vi "Do.vi"(8 "error in (no error)":errorcluster, 10 "Actor in":refnum<class "Actor.lvclass">, 11 "Connection Msg":refnum<class "Connection Msg.lvclass">) -> (0 "error out":errorcluster, 2 "Actor out":refnum<class "Actor.lvclass">)   [LabVIEW 2025, in "PLC_Abstr.lvlib" / "Connection Msg.lvclass"]
doc: "This VI delivers the message to the actor by calling the appropriate method(s) on the actor."
uses:
  Connection Msg.lvclass
  <vilib>/ActorFramework/Actor/Actor.lvclass
  Connection Msg.lvclass/Connection Msg.ctl
  PLC_Abstr/PLC_Abstr.lvclass
  9ef47adc-f318-494c-9b8b-6df3216d6863.vi
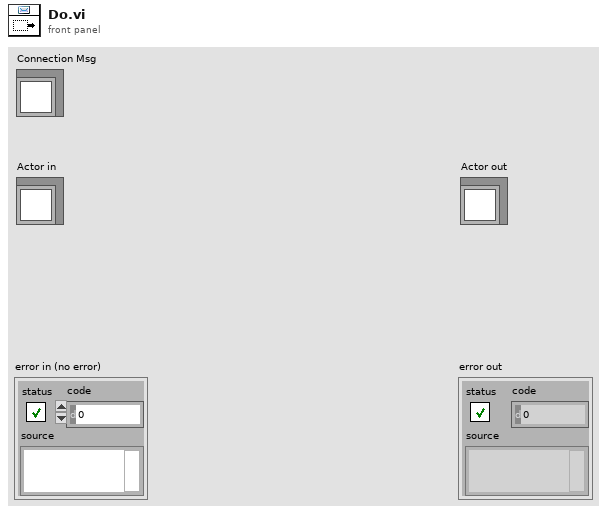
[diagram p1: front panel]
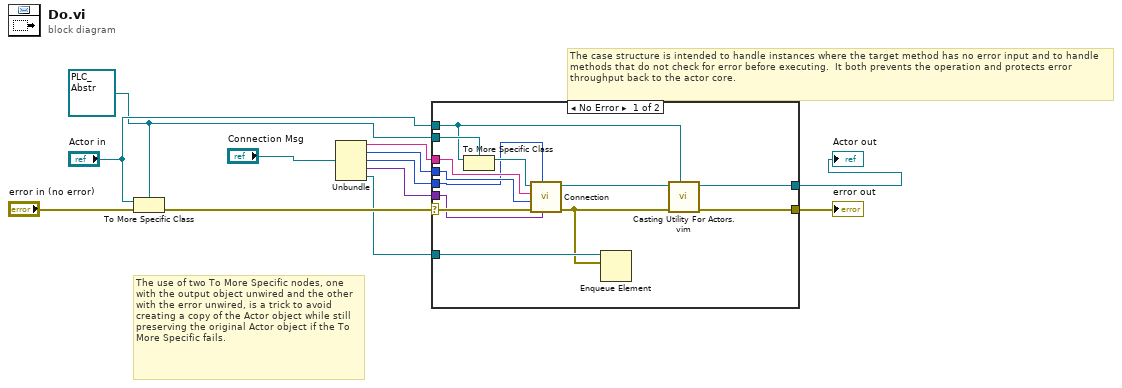
[diagram p0: block diagram]
diagram:
  w6 = refnum<class "PLC_Abstr.lvclass"> refnum ("Actor in")
  # "The use of two To More Specific nodes, one with the output object unwired and the other with the error unwired, is a trick to avoid creating a copy of the Actor object while still preserving the original Actor object if the To More Specific fails."
  # "The case structure is intended to handle instances where the target method has no error input and to handle methods that do not check for error before executing.  It both prevents the operation and protects error throughput back to the actor core."
  n1 = To More Specific Class(target class=w6, reference="Actor in", error in="error in (no error)") -> (error out=w10:errorcluster)  [unwired: 1 out]
  n2 = Unbundle("Connection Msg") -> (w5:string, w4:u16, w3:i32, w2:variant, w1:refnum<queue>)
  n3 = case shown="No Error" w10 {
    selector: w10 -> [w25 w27]
    tunnel: [w19 w27] -> w9
    tunnel: [w20 w26] -> w8
    tunnel: "Actor in" -> [w22 w26]
    tunnel: w6 -> [w23 _]
    tunnel: w5 -> [w18 _]
    tunnel: w4 -> [w17 _]
    tunnel: w3 -> [w16 _]
    tunnel: w2 -> [w15 _]
    tunnel: w1 -> [w14 _]
    frame No Error {
      n4 = To More Specific Class(target class=w23, reference=w22) -> (specific class reference=w24:refnum<class "PLC_Abstr.lvclass">)  [unwired: 1 in, 1 out]
      n5 = call-dynamic "Connection.vi"("Parameters"=w15, "Timeout"=w16, "error in (no error)"=w25, "Port"=w17, "IP Address"=w18, "PLC_Abstr in"=w24) -> ("error out"=w13:errorcluster, "PLC_Abstr out"=w21:refnum<class "PLC_Abstr.lvclass">)  [unwired: 4 in]
      n6 = Enqueue Element(queue=w14, element=w13) -> ()  [unwired: 2 in, 3 out]
      n7 = call "Casting Utility For Actors.vim"("type"=w22, "error in (no error)"=w13, "Actor in"=w21) -> ("error out"=w19:errorcluster, "Actor out"=w20:refnum<class "Actor.lvclass">)  [unwired: 7 in]
    }
    frame Error {
      # "If type check fails, pass the original object out again."
    }
  }
  "error out" <- w9
  "Actor out" <- w8
